vi "Get_length_of_Return.vi"(1 "Input string":string, 2 "Second variable name":string, 3 "First variable name":string) -> (0 "length":i32)   [LabVIEW 2011]
uses:
  Globals/Meas_global.vi
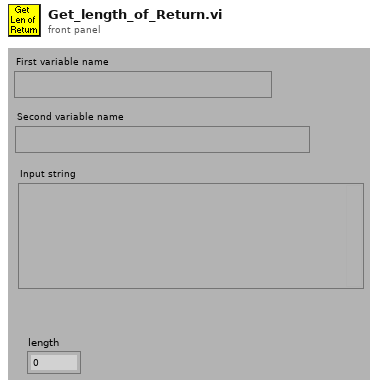
[diagram p1: front panel]
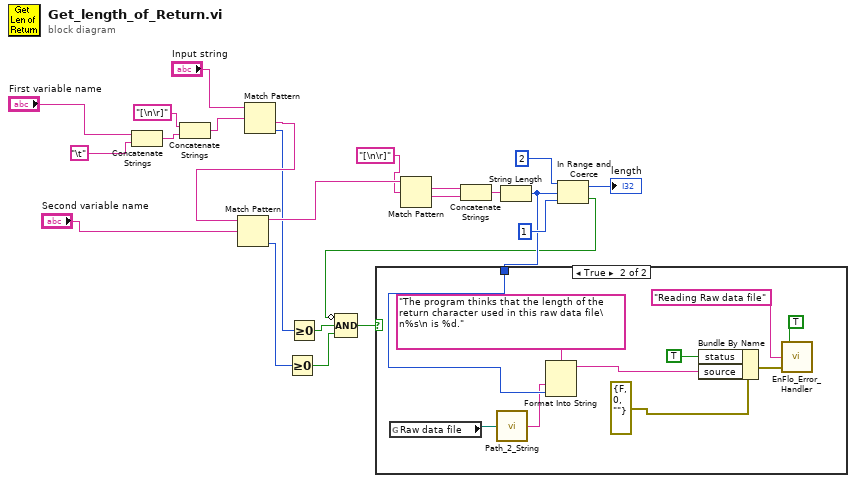
[diagram p0: block diagram]
diagram:
  n1 = Concatenate Strings("First variable name", "\t") -> (w20:string)
  n2 = Concatenate Strings("[\n\r]" ("x"), w20) -> (w19:string)
  n3 = Match Pattern(string="Input string", regular expression=w19) -> (after substring=w11:string, offset past match=w6:i32)  [unwired: 3 out]
  n4 = Match Pattern(string=w11, regular expression="Second variable name") -> (before substring=w17:string, offset past match=w5:i32)  [unwired: 3 out]
  n5 = Greater Or Equal To 0?(x=w5) -> (x >= 0?=w3:bool)
  n6 = Greater Or Equal To 0?(x=w6) -> (x >= 0?=w4:bool)
  n7 = Match Pattern(string=w17, regular expression="[\n\r]" ("x")) -> (match substring=w15:string, after substring=w14:string)  [unwired: 3 out]
  n8 = Concatenate Strings(w15, w14) -> (w13:string)
  n9 = String Length(string=w13) -> (length=w7:i32)
  n10 = In Range and Coerce(upper limit=2, x=w7, lower limit=1) -> (coerced(x)=→"length":i32, In Range?=w2:bool)
  n11 = Compound Arithmetic op=AND(invert w2, w4, w3) -> (w1:bool)
  n12 = case shown="True" w1 {
    tunnel: w7 -> [_ w26]
    frame False {
    }
    frame True {
      n13 = global read "Meas_global.vi" "Raw data file"() -> (w25:path)
      n14 = call "Path_2_String.vi"("Real Path"=w25) -> ("Path String"=w24:string)
      n15 = Format Into String(format string="The program thinks that the length of the return character used in this raw data file\n%s\n is %d." ("source"), w24, w26) -> (resulting string=w27:string)  [unwired: 2 in, 1 out]
      n16 = Bundle By Name(cluster=errorcluster {"status"=FALSE, "code"=0, "source"=""} ("error in (no error)"), "status"=TRUE, "source"=w27) -> (w31:errorcluster)
      n17 = call "EnFlo_Error_Handler.vi"("error in (no error)"=w31, "Error Type"="Reading Raw data file", "Dialog Box (T)"=TRUE) -> ()  [unwired: 3 out]
    }
  }
